vi "Set Temperature.vi"(8 "error in (no error)":errorcluster, 10 "Temp":i32, 11 "UV-VIS in":refnum<class "UV-VIS.lvclass">) -> (0 "error out":errorcluster, 3 "UV-VIS out":refnum<class "UV-VIS.lvclass">)   [LabVIEW 2015, in "UV-VIS.lvclass"]
uses:
  UV-VIS.lvclass
  Detector.lvclass/Detector.ctl
  GeneralFunctionality/GeneralFunctionality.lvclass/GeneralFunctionality.ctl
  Config/Config.lvclass
  Detector.lvclass
  GeneralFunctionality/GeneralFunctionality.lvclass
panel:
  out "DLL error code":u32
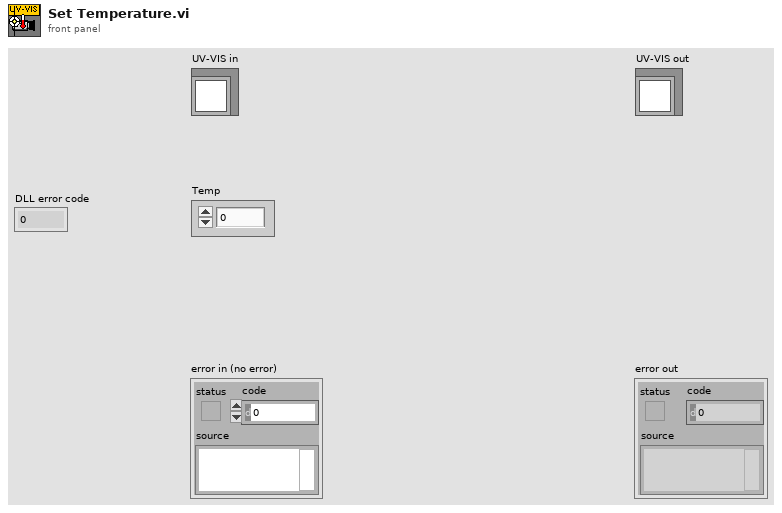
[diagram p1: front panel]
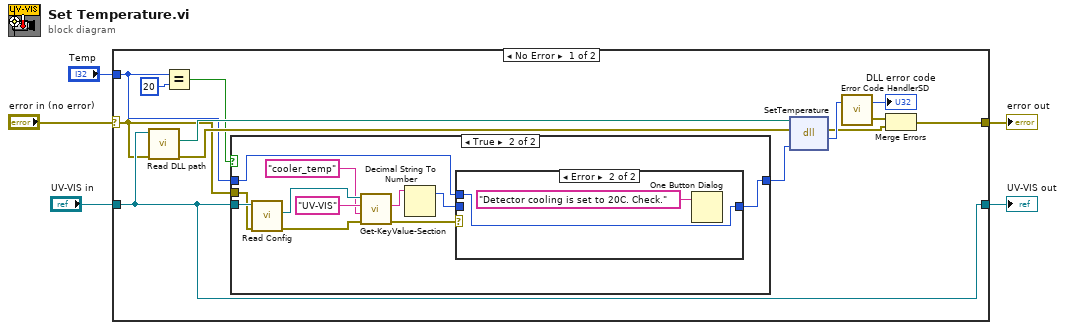
[diagram p0: block diagram]
diagram:
  n1 = case shown="No Error" "error in (no error)" {
    selector: "error in (no error)" -> [w8 w35]
    tunnel: [w12 w35] -> w3
    tunnel: [w9 w34] -> w4
    tunnel: "UV-VIS in" -> [w9 w34]
    tunnel: "Temp" -> [w6 _]
    frame No Error {
      n2 = call "Read DLL path.vi"("error in (no error)"=w8, "Detector in"=w9) -> ("error out"=w15:errorcluster, "DLL path"=w16:path)  [unwired: 7 in, 1 out]
      n3 = Equal?(x=w6, y=20) -> (x = y?=w10:bool)
      n4 = case shown="True" w10 {
        tunnel: w9 -> [_ w26]
        tunnel: w8 -> [_ w24]
        tunnel: [w19 w21] -> w7
        tunnel: w6 -> [w19 w20]
        frame False {
        }
        frame True {
          n5 = call "Read Config.vi"("error in (no error)"=w24, "GeneralFunctionality en entrée"=w26) -> ("error out"=w25:errorcluster, "Config.lvclass"=w30:refnum<class "Config.lvclass">)  [unwired: 7 in, 1 out]
          n6 = call-dynamic "Get-KeyValue-Section.vi"("error in (no error)"=w25, "Key"="cooler_temp", "Section"="UV-VIS", "Config in"=w30) -> ("error out"=w23:errorcluster, "Value"=w27:string)  [unwired: 5 in, 1 out]
          n7 = Decimal String To Number(string=w27) -> (offset past number=w22:i32)  [unwired: 2 in, 1 out]
          n8 = case shown="Error" w23 {
            tunnel: w22 -> [w31 _]
            tunnel: [w31 w33] -> w21
            tunnel: w20 -> [_ w33]
            frame No Error {
            }
            frame Error {
              n9 = One Button Dialog(message="Detector cooling is set to 20C. Check.") -> ()  [unwired: 1 in, 1 out]
            }
          }
        }
      }
      n10 = dll-call lib="S:/TRANCON/DLL/Atmcd32d.dll" fn="SetTemperature"(path in=w16, error in=w15, "temperature"=w7) -> (error out=w14:errorcluster, "return type"=w18:u32)  [unwired: 2 in, 1 out]
      n11 = call "Error Code HandlerSD.vi"("DLL error code"=w18) -> ("error out"=w13:errorcluster, "dup DLL error code"=→"DLL error code":u32)  [unwired: 1 in]
      n12 = Merge Errors(w13, w14) -> (w12:errorcluster)
    }
    frame Error {
    }
  }
  "error out" <- w3
  "UV-VIS out" <- w4
